vi "Begin.vi"(8 "error in":errorcluster) -> (0 "error out":errorcluster)   [LabVIEW 2019]
doc: "Called before other user functions, this VI is expected to open initial I/O refnums, load in file data, and do all program initialization. Notice that the <B>error out</B> terminal is simply used for data flow. Wiring it to other structures or subVIs ensures that this VI runs first."
uses:
  <vilib>/Rock Robotics/SystemInterfaces/i2clib/i2c_bus.ctl
  <vilib>/Rock Robotics/WPI/DriverStation/WPI_DriverStationRobotMode2.ctl
  <vilib>/Rock Robotics/WPI/Joystick/WPI_JoystickDeviceEnum.ctl
  <vilib>/Rock Robotics/WPI/Solenoid/WPI_SolenoidChannel.ctl
  <vilib>/Rock Robotics/WPI/SafetyOutput/WPI_SafetyOutputConfigMenu.ctl
  <vilib>/Rock Robotics/WPI/ThirdParty/REV Robotics/SPARK MAX/Typedef/Spark MAX Motor Type.ctl
  <vilib>/Rock Robotics/WPI/ThirdParty/REV Robotics/SPARK MAX/Typedef/Spark MAX Sensor Type.ctl
  <vilib>/Rock Robotics/SystemInterfaces/DIO/FPGA_DIOChannel.ctl
  <vilib>/Rock Robotics/SystemInterfaces/DIO/FPGA_DIOPWMChannel.ctl
  Robot Global Data.vi
  <vilib>/Rock Robotics/Network Tables/NT Write String Array.vi
  <vilib>/Rock Robotics/WPI/RobotDrive/WPI_RobotDriveOpen2MotorWithExistingMotors.vi
  <vilib>/Rock Robotics/WPI/Solenoid/WPI_SolenoidOpenDouble.vi
  <vilib>/Rock Robotics/WPI/MotorControl/WPI_MotorControlOpen SPARK.vi
  <vilib>/Rock Robotics/WPI/RobotDrive/WPI_RobotDriveOpen2MotorWithVictorSPX.vi
  <vilib>/Rock Robotics/SystemInterfaces/spilib/spi_bus.ctl
  <vilib>/Rock Robotics/WPI/Gyro/WPI_GyroXRS450_SPI_Open.vi
panel:
  out "String":string="Velocity Tune"
  out "String 2":string="Smart Motion Tune"
  out "String 3":string="Tuning Instructions:\n\n0) Before using this function, you should understand from your specific mechanism the max acceleration and the max velocity. You can obtain these either by design constraints, or running in open loop mode and calculating these values.\n\n1) Set the 'Mode' switch to 'Velocity Tune'\n\n2) Tune the mechanism as you would a Velocity PID loop until the mechanism is controlled fairly well. In this mode the Setpoint slider controls the Velocity of the mechanism.\n\n3) Configure the smart motion parameters, and set the 'Mode' switch to 'Smart Motion'. In this mode, the Setpoint slider controls the Position of the mechansim. For initial tests it is recommended to keep the max velocity and max acceleration lower than the max value, and slowly increase these to the desired level.\n\n4) Test the mechanism by setting the position within the allowable range of the mechanism, and slowly increase limits until the system is working as intended."
  in  "I2C Bus":T1
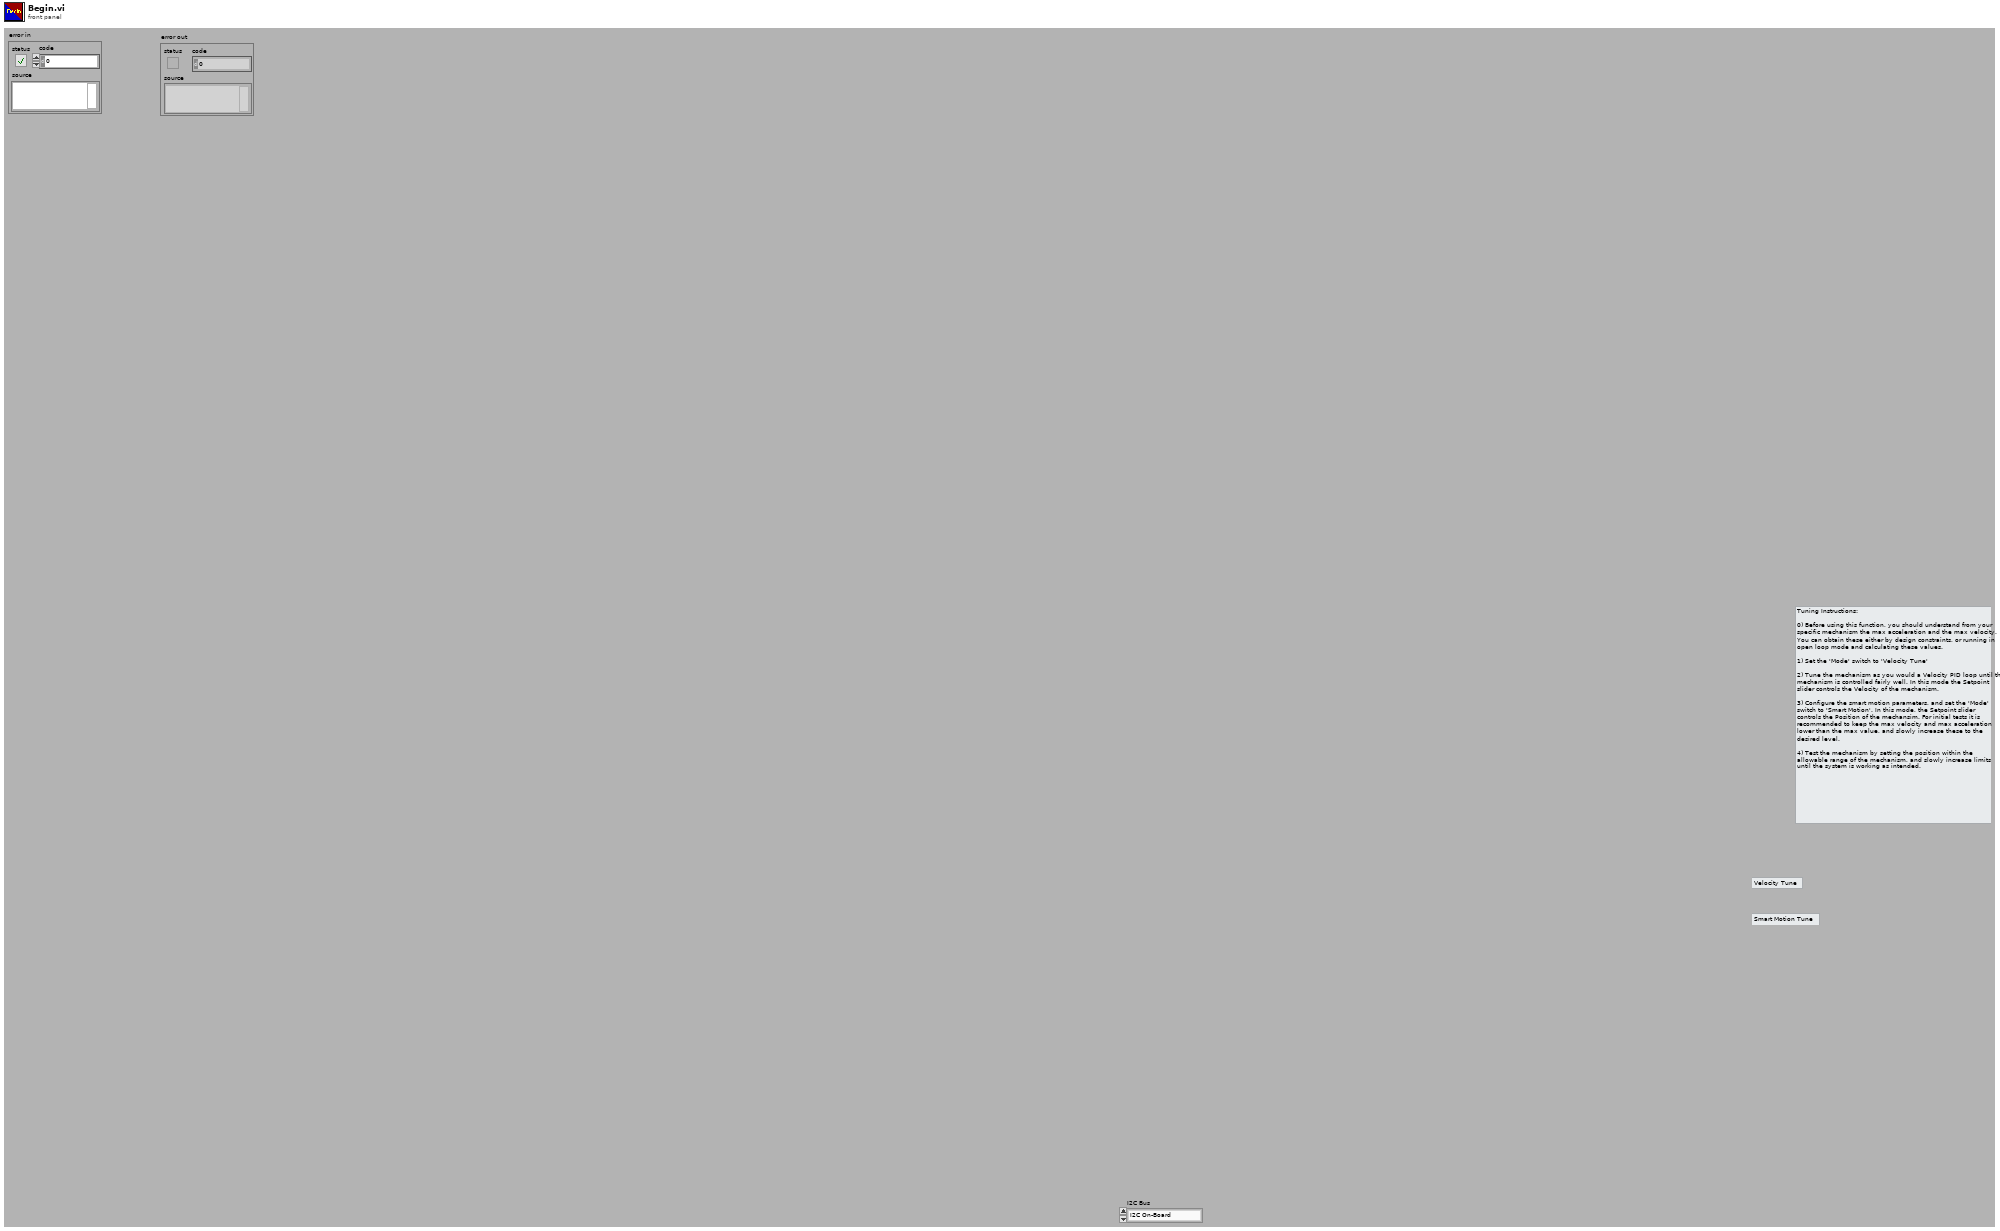
[diagram p1: front panel]
types:
  T1 = typedef "i2c_bus.ctl" = enum16{"I2C On-Board", "I2C MXP", "Invalid"}
  T2 = typedef "FPGA_DIOPWMChannel.ctl" = enum8{"PWM 0", "PWM 1", "PWM 2", "PWM 3", "PWM 4", "PWM 5", "PWM 6", "PWM 7", "PWM 8", "PWM 9", "PWM MXP 0", "PWM MXP 1", "PWM MXP 2", "PWM MXP 3", "PWM MXP 4", "PWM MXP 5", "PWM MXP 6", "PWM MXP 7", "PWM MXP 8", "PWM MXP 9", "Invalid"}
  T3 = typedef "WPI_SafetyOutputConfigMenu.ctl" = enum16{"Enable", "Disable"}
  T4 = typedef "WPI_SolenoidChannel.ctl" = enum8{"Solenoid 0", "Solenoid 1", "Solenoid 2", "Solenoid 3", "Solenoid 4", "Solenoid 5", "Solenoid 6", "Solenoid 7", "Invalid"}
  T5 = typedef "FPGA_DIOChannel.ctl" = enum8{"DIO 0", "DIO 1", "DIO 2", "DIO 3", "DIO 4", "DIO 5", "DIO 6", "DIO 7", "DIO 8", "DIO 9", "DIO MXP 0", "DIO MXP 1", "DIO MXP 2", "DIO MXP 3", "DIO MXP 4", "DIO MXP 5", "DIO MXP 6", "DIO MXP 7", "DIO MXP 8", "DIO MXP 9", "DIO MXP 10", "DIO MXP 11", "DIO MXP 12", "DIO MXP 13", "DIO MXP 14", "DIO MXP 15", "SPI Port CS1", "SPI Port CS2", "SPI Port CS3", "SPI Port MISO", "SPI Port MOSI", "Invalid"}
  T6 = typedef "Spark MAX Sensor Type.ctl" = enum16{"No Sensor", "Hall Sensor", "Encoder", "-Not Available-", "Analog", "Alternate Encoder"}
  T7 = typedef "Spark MAX Motor Type.ctl" = enum16{"Brushed", "Brushless"}
  T8 = typedef "WPI_JoystickDeviceEnum.ctl" = enum16{"USB 0", "USB 1", "USB 2", "USB 3", "USB 4", "USB 5"}
  T9 = typedef "WPI_DriverStationRobotMode2.ctl" = enum16{"Autonomous Disabled", "Autonomous Enabled", "Teleop Disabled", "Teleop Enabled", "Disconnected", "Finish", "Test Disabled", "Test Enabled", "Emergency Stopped"}
  T10 = typedef "WPI_MotorControlDeviceRef.ctl" = cluster{"DeviceStatus":errorcluster, "Type":T11, "PWM":cluster{"PWM Channel":T2, "DeadBand":T12}, "CAN":cluster{"Device Number":u8, "SetOutput VI Ref":variant, "GetOutput VI Ref":variant, "Enable VI Ref":variant, "Disable VI Ref":variant, "Data":variant}, "Invert":bool, "DIO PWM":cluster{"PWM \"Enable\" Channel":T2, "DIOChannel":T5, "PWM Rate":dbl}}
  T11 = typedef "WPI_MotorControlType.ctl" = enum16{"PWM", "CAN", "DIO PWM"}
  T12 = typedef "WPI_PWMDeadband.ctl" = cluster{"Name":string, "maxPositivePwm":i32, "minPositivePwm":i32, "centerPwm":i32, "maxNegativePwm":i32, "minNegativePwm":i32, "angularRange":u16}
  T13 = typedef "WPI_JoystickDevRef.ctl" = cluster{"Device":T8}
  T14 = typedef "WPI_RobotDriveDevRef.ctl" = cluster{"DevStatus":errorcluster, "Motors[]":T10[], "Square Inputs":bool, "Max Output":dbl}
  T15 = typedef "WPI_DigitalInputDevRef.ctl" = cluster{"DevStatus":errorcluster, "DIO Channel":T5}
  T16 = typedef "spi_bus.ctl" = enum16{"SPI On-Board, CS0", "SPI On-Board, CS1", "SPI On-Board, CS2", "SPI On-Board, CS3", "SPI MXP", "Invalid"}
  T17 = typedef "WPI_GyroDevRef.ctl" = cluster{"DevStatus":errorcluster, "Analog Channel":T18, "Gain (VoltsPerDegree/Second)":dbl, "Gyro Type":enum16{"Analog", "XRS450"}, "Handle":i32, "SPI Bus":T16, "Device Found":bool, "Sample Rate":dbl, "Calibrate On Open":bool, "Offset":dbl}
  T18 = typedef "FPGA_AIChannel.ctl" = enum8{"AI 0", "AI 1", "AI 2", "AI 3", "AI MXP 0", "AI MXP 1", "AI MXP 2", "AI MXP 3", "Invalid"}
  T19 = typedef "Color Sensor V3 DevRef.ctl" = cluster{"I2CDevRef":T20}
  T20 = typedef "WPI_I2CDevRef.ctl" = cluster{"DevStatus":errorcluster, "Device Address":u8, "Handle":i32, "I2C Bus":T1}
  T21 = typedef "WPI_SolenoidDevRef.ctl" = cluster{"DevStatus":errorcluster, "Pneumatics Control Module":u8, "Forward Solenoid Channel":T4, "Reverse Solenoid Channel":T4}
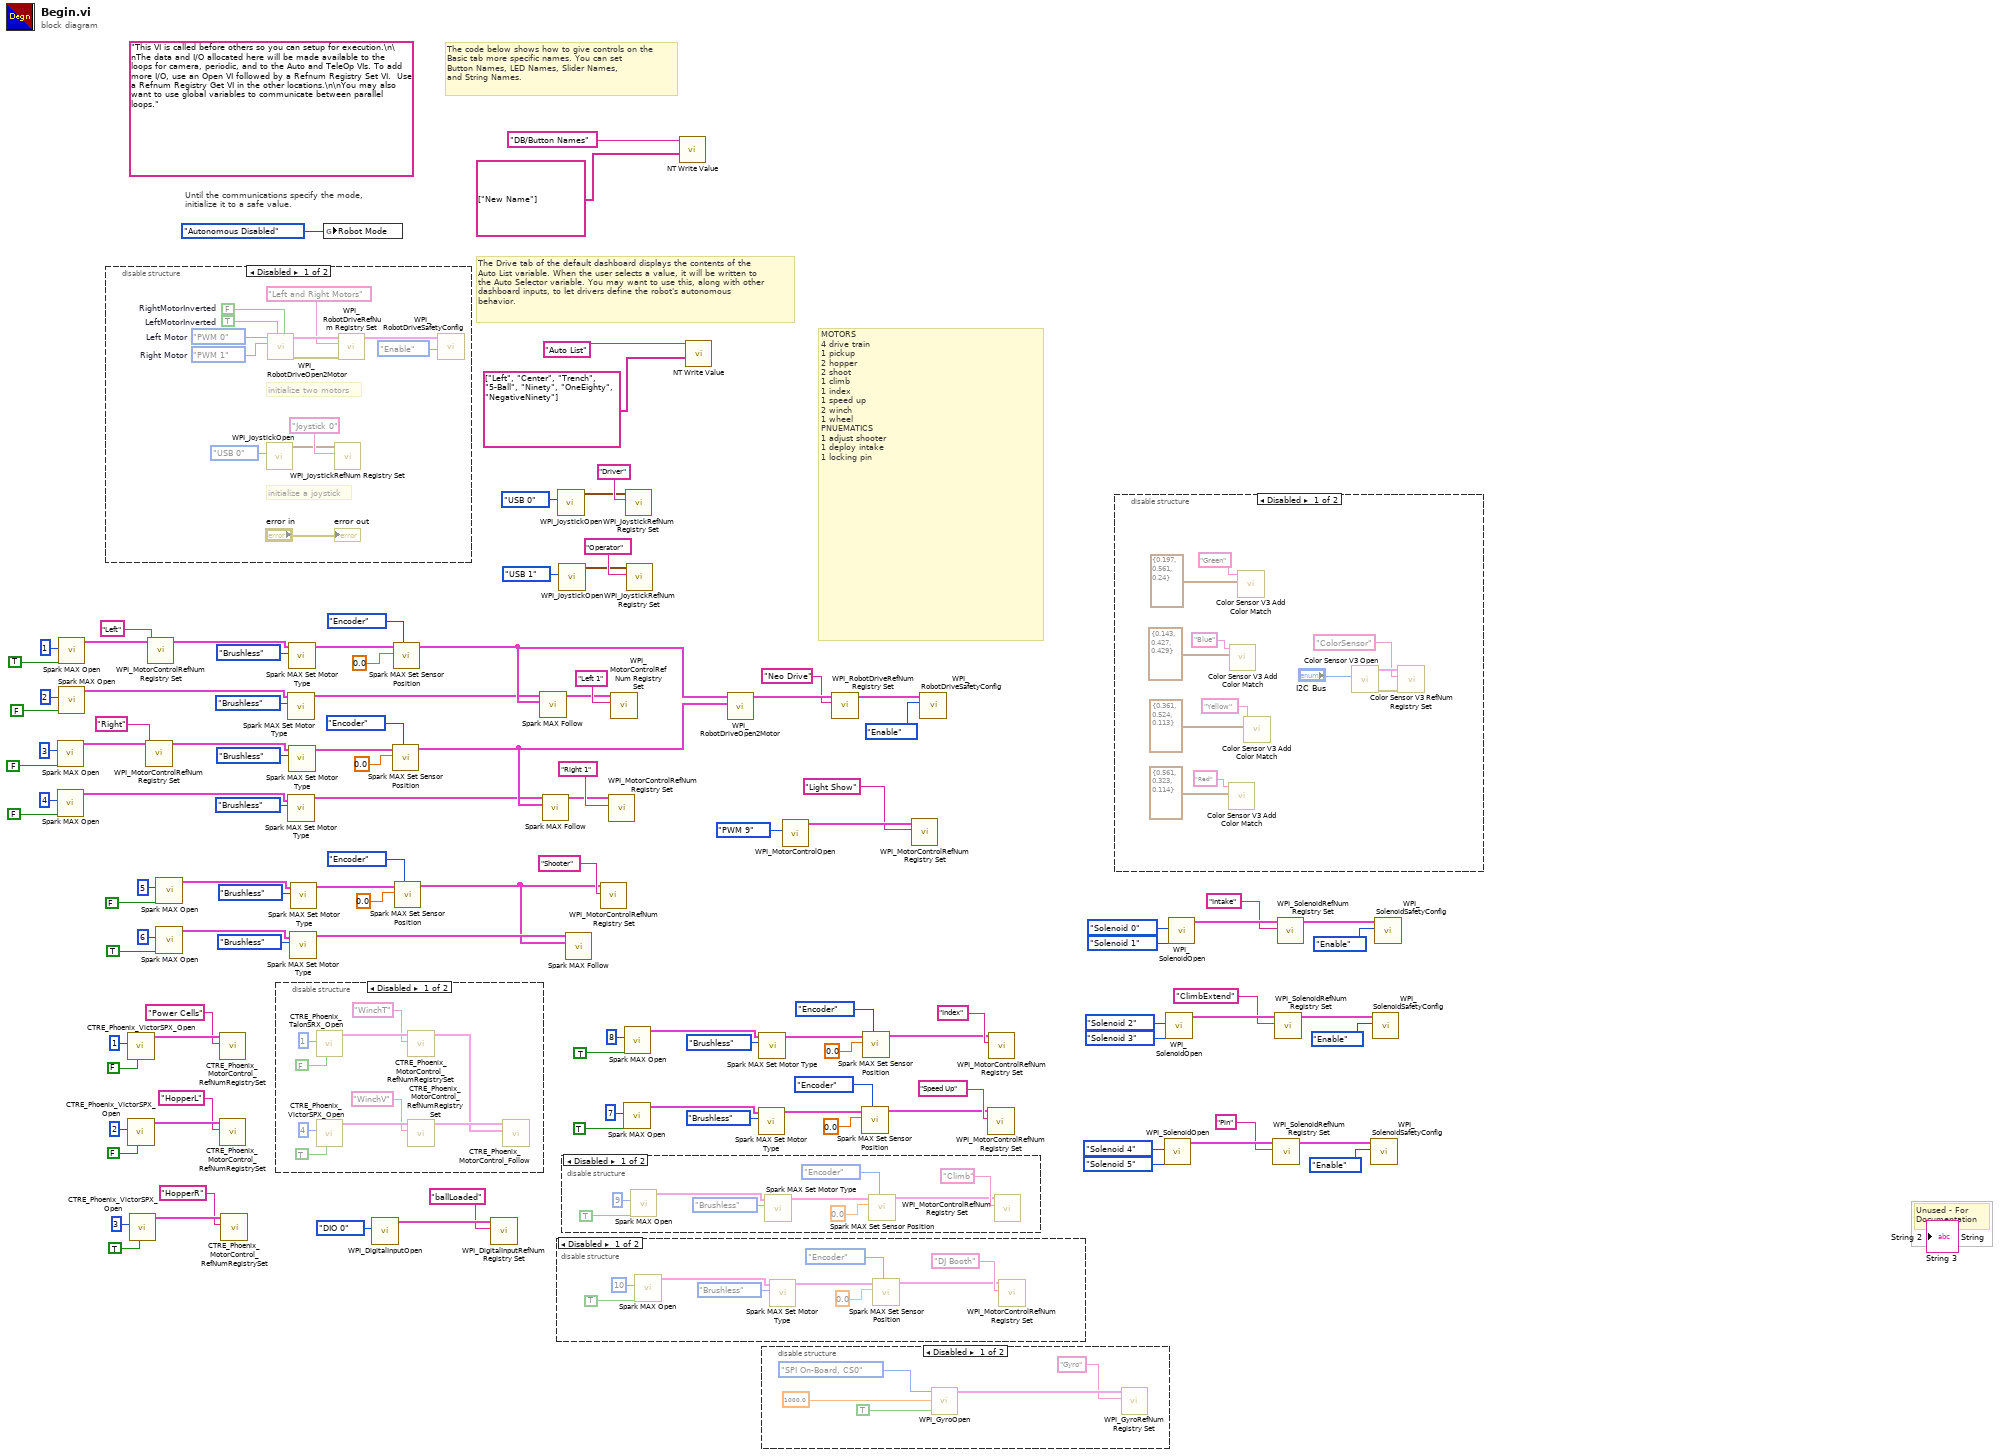
[diagram p0: block diagram]
diagram:
  (unwired) "This VI is called before others so you can setup for execution.\n\nThe data and I/O allocated here will be made available to the loops for camera, periodic, and to the Auto and TeleOp VIs. To add more I/O, use an Open VI followed by a Refnum Registry Set VI.  Use a Refnum Registry Get VI in the other locations.\n\nYou may also want to use global variables to communicate between parallel loops."
  # "Unused - For Documentation"
  # "MOTORS\n4 drive train\n1 pickup\n2 hopper\n2 shoot\n1 climb\n1 index\n1 speed up\n2 winch\n1 wheel\nPNUEMATICS\n1 adjust shooter\n1 deploy intake\n1 locking pin"
  # "The Drive tab of the default dashboard displays the contents of the\nAuto List variable. When the user selects a value, it will be written to\nthe Auto Selector variable. You may want to use this, along with other\ndashboard inputs, to let drivers define the robot's autonomous\nbehavior."
  # "The code below shows how to give controls on the\nBasic tab more specific names. You can set\nButton Names, LED Names, Slider Names,\nand String Names."
  # "Until the communications specify the mode,\ninitialize it to a safe value."
  n1 = call <vilib>:"Spark MAX Open.vi"("Invert"=FALSE, "Device Number"=u8 3) -> ("MotorControlDeviceRef"=w59:T10)  [unwired: 8 in, 1 out]
  n2 = call <vilib>:"Spark MAX Open.vi"("Invert"=FALSE, "Device Number"=u8 4) -> ("MotorControlDeviceRef"=w93:T10)  [unwired: 8 in, 1 out]
  n3 = call <vilib>:"Spark MAX Open.vi"("Invert"=TRUE, "Device Number"=u8 1) -> ("MotorControlDeviceRef"=w62:T10)  [unwired: 8 in, 1 out]
  n4 = call <vilib>:"Spark MAX Open.vi"("Invert"=FALSE, "Device Number"=u8 2) -> ("MotorControlDeviceRef"=w94:T10)  [unwired: 8 in, 1 out]
  n5 = disable-structure shown="Disabled" {
    frame Disabled {
      w124 = FPGA_DIOPWMChannel."PWM 1"  # Right Motor
      w125 = FPGA_DIOPWMChannel."PWM 0"  # Left Motor
      w129 = TRUE  # LeftMotorInverted
      w130 = FALSE  # RightMotorInverted
      # "initialize a joystick"
      # "initialize two motors"
      n6 = call <vilib>:"WPI_JoystickOpen.vi"("JoystickDevice"=WPI_JoystickDeviceEnum."USB 0") -> ("JoystickDevRef"=w120:T13)  [unwired: 10 in]
      n7 = call-poly <vilib>:"WPI_RobotDriveOpen2Motor.vi"("Right Motor Inverted"=w130, "Left Motor Inverted"=w129, "Right Motor"=w124, "Left Motor"=w125) -> ("error out"=w126:errorcluster, "RobotDriveDevRef"=w128:T14)  [unwired: 1 in, 5 out]
      n8 = call <vilib>:"WPI_JoystickRefNum Registry Set.vi"("refnum name"="Joystick 0", "JoystickDevRef"=w120) -> ()  [unwired: 8 in, 2 out]
      n9 = call <vilib>:"WPI_RobotDriveRefNum Registry Set.vi"("error in (no error)"=w126, "refnum name"="Left and Right Motors", "RobotDriveDevRef"=w128) -> ("RobotDriveDevRef"=w123:T14)  [unwired: 1 in, 7 out]
      n10 = call <vilib>:"WPI_RobotDriveSafetyConfig.vi"("mode"=WPI_SafetyOutputConfigMenu."Enable", "RobotDriveDevRef"=w123) -> ()  [unwired: 8 in, 2 out]
      "error out" <- "error in"
    }
    frame Enabled {
    }
  }
  n11 = call <vilib>:"CTRE_Phoenix_VictorSPX_Open.vi"("Invert"=FALSE, "Device Number"=u8 1) -> ("CAN Talon SRX Ref"=w49:T10)  [unwired: 8 in, 1 out]
  n12 = call <vilib>:"CTRE_Phoenix_VictorSPX_Open.vi"("Invert"=FALSE, "Device Number"=u8 2) -> ("CAN Talon SRX Ref"=w42:T10)  [unwired: 8 in, 1 out]
  n13 = call <vilib>:"CTRE_Phoenix_VictorSPX_Open.vi"("Invert"=TRUE, "Device Number"=u8 3) -> ("CAN Talon SRX Ref"=w45:T10)  [unwired: 8 in, 1 out]
  n14 = call <vilib>:"WPI_MotorControlRefNum Registry Set.vi"("refnum name"="Right", "MotorControlDevRef"=w59) -> ("MotorControlDevRef"=w57:T10)  [unwired: 8 in, 1 out]
  n15 = call <vilib>:"WPI_MotorControlRefNum Registry Set.vi"("refnum name"="Left", "MotorControlDevRef"=w62) -> ("MotorControlDevRef"=w60:T10)  [unwired: 8 in, 1 out]
  n16 = call <vilib>:"Spark MAX Open.vi"("Invert"=FALSE, "Device Number"=u8 5) -> ("MotorControlDeviceRef"=w74:T10)  [unwired: 8 in, 1 out]
  n17 = call <vilib>:"Spark MAX Open.vi"("Invert"=TRUE, "Device Number"=u8 6) -> ("MotorControlDeviceRef"=w73:T10)  [unwired: 8 in, 1 out]
  n18 = call <vilib>:"CTRE_Phoenix_MotorControl_RefNumRegistrySet.vi"("refnum name"="Power Cells", "PhoenixMotorControlDevRef"=w49) -> ()  [unwired: 8 in, 2 out]
  n19 = call <vilib>:"CTRE_Phoenix_MotorControl_RefNumRegistrySet.vi"("refnum name"="HopperL", "PhoenixMotorControlDevRef"=w42) -> ()  [unwired: 8 in, 2 out]
  n20 = call <vilib>:"CTRE_Phoenix_MotorControl_RefNumRegistrySet.vi"("refnum name"="HopperR", "PhoenixMotorControlDevRef"=w45) -> ()  [unwired: 8 in, 2 out]
  n21 = disable-structure shown="Disabled" {
    frame Disabled {
      n22 = call <vilib>:"CTRE_Phoenix_TalonSRX_Open.vi"("Invert"=FALSE, "Device Number"=u8 1) -> ("CAN Talon SRX Ref"=w135:T10)  [unwired: 8 in, 1 out]
      n23 = call <vilib>:"CTRE_Phoenix_VictorSPX_Open.vi"("Invert"=TRUE, "Device Number"=u8 4) -> ("CAN Talon SRX Ref"=w139:T10)  [unwired: 8 in, 1 out]
      n24 = call <vilib>:"CTRE_Phoenix_MotorControl_RefNumRegistrySet.vi"("refnum name"="WinchT", "PhoenixMotorControlDevRef"=w135) -> ("PhoenixMotorControlDevRef"=w131:T10)  [unwired: 8 in, 1 out]
      n25 = call <vilib>:"CTRE_Phoenix_MotorControl_RefNumRegistrySet.vi"("refnum name"="WinchV", "PhoenixMotorControlDevRef"=w139) -> ("PhoenixMotorControlDevRef"=w132:T10)  [unwired: 8 in, 1 out]
      n26 = call <vilib>:"CTRE_Phoenix_MotorControl_Follow.vi"("Master Controller to Follow"=w131, "PhoenixMotorControlDevRef"=w132) -> ()  [unwired: 8 in, 2 out]
    }
    frame Enabled {
    }
  }
  n27 = call <vilib>:"Spark MAX Set Motor Type.vi"("Motor Type"=Spark_MAX_Motor_Type."Brushless", "MotorControlDevRef"=w94) -> ("MotorControlDeviceRef"=w63:T10)  [unwired: 8 in, 1 out]
  n28 = call <vilib>:"Spark MAX Set Motor Type.vi"("Motor Type"=Spark_MAX_Motor_Type."Brushless", "MotorControlDevRef"=w93) -> ("MotorControlDeviceRef"=w66:T10)  [unwired: 8 in, 1 out]
  n29 = call <vilib>:"Spark MAX Set Motor Type.vi"("Motor Type"=Spark_MAX_Motor_Type."Brushless", "MotorControlDevRef"=w60) -> ("MotorControlDeviceRef"=w88:T10)  [unwired: 8 in, 1 out]
  n30 = call <vilib>:"Spark MAX Set Motor Type.vi"("Motor Type"=Spark_MAX_Motor_Type."Brushless", "MotorControlDevRef"=w57) -> ("MotorControlDeviceRef"=w89:T10)  [unwired: 8 in, 1 out]
  n31 = call <vilib>:"Spark MAX Set Motor Type.vi"("Motor Type"=Spark_MAX_Motor_Type."Brushless", "MotorControlDevRef"=w73) -> ("MotorControlDeviceRef"=w20:T10)  [unwired: 8 in, 1 out]
  n32 = call <vilib>:"Spark MAX Set Motor Type.vi"("Motor Type"=Spark_MAX_Motor_Type."Brushless", "MotorControlDevRef"=w74) -> ("MotorControlDeviceRef"=w71:T10)  [unwired: 8 in, 1 out]
  n33 = global write "Robot Global Data.vi" "Robot Mode"(WPI_DriverStationRobotMode2."Autonomous Disabled" ("Robot Mode")) -> ()
  n34 = call <vilib>:"WPI_DigitalInputOpen.vi"("DIO Channel"=FPGA_DIOChannel."DIO 0") -> ("DigitalInputDevRef"=w17:T15)  [unwired: 9 in, 1 out]
  n35 = call <vilib>:"Spark MAX Set Sensor Position.vi"("Sensor Type (Hall Sensor)"=Spark_MAX_Sensor_Type."Encoder", "Position"=0.0, "MotorControlDeviceRef"=w89) -> ("MotorControlDeviceRef"=w67:T10)  [unwired: 7 in, 1 out]
  n36 = call <vilib>:"Spark MAX Set Sensor Position.vi"("Sensor Type (Hall Sensor)"=Spark_MAX_Sensor_Type."Encoder", "Position"=0.0, "MotorControlDeviceRef"=w88) -> ("MotorControlDeviceRef"=w64:T10)  [unwired: 7 in, 1 out]
  n37 = call <vilib>:"Spark MAX Set Sensor Position.vi"("Sensor Type (Hall Sensor)"=Spark_MAX_Sensor_Type."Encoder", "Position"=0.0, "MotorControlDeviceRef"=w71) -> ("MotorControlDeviceRef"=w19:T10)  [unwired: 7 in, 1 out]
  n38 = call <vilib>:"WPI_DigitalInputRefNum Registry Set.vi"("refnum name"="ballLoaded", "DigitalInputDevRef"=w17) -> ()  [unwired: 8 in, 2 out]
  n39 = call <vilib>:"Spark MAX Follow.vi"("Master Controller"=w64, "MotorControlDeviceRef"=w63) -> ("MotorControlDeviceRef"=w65:T10)  [unwired: 8 in, 1 out]
  n40 = call <vilib>:"Spark MAX Follow.vi"("Master Controller"=w67, "MotorControlDeviceRef"=w66) -> ("MotorControlDeviceRef"=w68:T10)  [unwired: 8 in, 1 out]
  n41 = disable-structure shown="Disabled" {
    frame Disabled {
      n42 = call <vilib>:"Spark MAX Open.vi"("Invert"=TRUE, "Device Number"=u8 10) -> ("MotorControlDeviceRef"=w146:T10)  [unwired: 8 in, 1 out]
      n43 = call <vilib>:"Spark MAX Set Motor Type.vi"("Motor Type"=Spark_MAX_Motor_Type."Brushless", "MotorControlDevRef"=w146) -> ("MotorControlDeviceRef"=w144:T10)  [unwired: 8 in, 1 out]
      n44 = call <vilib>:"Spark MAX Set Sensor Position.vi"("Sensor Type (Hall Sensor)"=Spark_MAX_Sensor_Type."Encoder", "Position"=0.0, "MotorControlDeviceRef"=w144) -> ("MotorControlDeviceRef"=w141:T10)  [unwired: 7 in, 1 out]
      n45 = call <vilib>:"WPI_MotorControlRefNum Registry Set.vi"("refnum name"="DJ Booth", "MotorControlDevRef"=w141) -> ()  [unwired: 8 in, 2 out]
    }
    frame Enabled {
    }
  }
  n46 = call <vilib>:"WPI_JoystickOpen.vi"("JoystickDevice"=WPI_JoystickDeviceEnum."USB 0") -> ("JoystickDevRef"=w111:T13)  [unwired: 10 in]
  n47 = call <vilib>:"WPI_JoystickOpen.vi"("JoystickDevice"=WPI_JoystickDeviceEnum."USB 1") -> ("JoystickDevRef"=w108:T13)  [unwired: 10 in]
  n48 = disable-structure shown="Disabled" {
    frame Disabled {
      n49 = call <vilib>:"Spark MAX Open.vi"("Invert"=TRUE, "Device Number"=u8 9) -> ("MotorControlDeviceRef"=w155:T10)  [unwired: 8 in, 1 out]
      n50 = call <vilib>:"Spark MAX Set Motor Type.vi"("Motor Type"=Spark_MAX_Motor_Type."Brushless", "MotorControlDevRef"=w155) -> ("MotorControlDeviceRef"=w153:T10)  [unwired: 8 in, 1 out]
      n51 = call <vilib>:"Spark MAX Set Sensor Position.vi"("Sensor Type (Hall Sensor)"=Spark_MAX_Sensor_Type."Encoder", "Position"=0.0, "MotorControlDeviceRef"=w153) -> ("MotorControlDeviceRef"=w150:T10)  [unwired: 7 in, 1 out]
      n52 = call <vilib>:"WPI_MotorControlRefNum Registry Set.vi"("refnum name"="Climb", "MotorControlDevRef"=w150) -> ()  [unwired: 8 in, 2 out]
    }
    frame Enabled {
    }
  }
  n53 = call <vilib>:"Spark MAX Follow.vi"("Master Controller"=w19, "MotorControlDeviceRef"=w20) -> ()  [unwired: 8 in, 2 out]
  n54 = call <vilib>:"WPI_MotorControlRefNum Registry Set.vi"("refnum name"="Shooter", "MotorControlDevRef"=w19) -> ()  [unwired: 8 in, 2 out]
  n55 = call <vilib>:"WPI_MotorControlRefNum Registry Set.vi"("refnum name"="Right 1", "MotorControlDevRef"=w68) -> ()  [unwired: 8 in, 2 out]
  n56 = call <vilib>:"WPI_MotorControlRefNum Registry Set.vi"("refnum name"="Left 1", "MotorControlDevRef"=w65) -> ()  [unwired: 8 in, 2 out]
  n57 = call <vilib>:"Spark MAX Open.vi"("Invert"=TRUE, "Device Number"=u8 7) -> ("MotorControlDeviceRef"=w35:T10)  [unwired: 8 in, 1 out]
  n58 = call <vilib>:"Spark MAX Open.vi"("Invert"=TRUE, "Device Number"=u8 8) -> ("MotorControlDeviceRef"=w26:T10)  [unwired: 8 in, 1 out]
  n59 = call <vilib>:"WPI_JoystickRefNum Registry Set.vi"("refnum name"="Driver", "JoystickDevRef"=w111) -> ()  [unwired: 8 in, 2 out]
  n60 = call <vilib>:"WPI_JoystickRefNum Registry Set.vi"("refnum name"="Operator", "JoystickDevRef"=w108) -> ()  [unwired: 8 in, 2 out]
  n61 = call-poly <vilib>:"NT Write Value.vi"("String Array"=string[] ["New Name"], "Name"="DB/Button Names") -> ()  [unwired: 9 in, 1 out]
  n62 = call-poly <vilib>:"NT Write Value.vi"("String Array"=string[] ["Left", "Center", "Trench", "5-Ball", "Ninety", "OneEighty", "NegativeNinety"], "Name"="Auto List") -> ()  [unwired: 9 in, 1 out]
  n63 = call-poly <vilib>:"WPI_RobotDriveOpen2Motor.vi"("Right Motor Dev Ref"=w67, "Left Motor Dev Ref"=w64) -> ("RobotDriveDevRef"=w84:T14)  [unwired: 8 in, 1 out]
  n64 = call <vilib>:"Spark MAX Set Motor Type.vi"("Motor Type"=Spark_MAX_Motor_Type."Brushless", "MotorControlDevRef"=w35) -> ("MotorControlDeviceRef"=w33:T10)  [unwired: 8 in, 1 out]
  n65 = call <vilib>:"Spark MAX Set Motor Type.vi"("Motor Type"=Spark_MAX_Motor_Type."Brushless", "MotorControlDevRef"=w26) -> ("MotorControlDeviceRef"=w24:T10)  [unwired: 8 in, 1 out]
  n66 = disable-structure shown="Disabled" {
    frame Disabled {
      n67 = call-poly <vilib>:"WPI_GyroOpen.vi"("Calibrate On Open"=TRUE, "Sample Rate (Hz)"=1000.0, "SPI Bus"=spi_bus."SPI On-Board, CS0") -> ("GyroDevRef"=w162:T17)  [unwired: 6 in, 2 out]
      n68 = call <vilib>:"WPI_GyroRefNum Registry Set.vi"("refnum name"="Gyro", "GyroDevRef"=w162) -> ()  [unwired: 8 in, 2 out]
    }
    frame Enabled {
    }
  }
  n69 = call-poly <vilib>:"WPI_MotorControlOpen.vi"("PWM Channel"=FPGA_DIOPWMChannel."PWM 9") -> ("MotorControlDeviceRef"=w2:T10)  [unwired: 9 in, 1 out]
  n70 = call <vilib>:"WPI_RobotDriveRefNum Registry Set.vi"("refnum name"="Neo Drive", "RobotDriveDevRef"=w84) -> ("RobotDriveDevRef"=w82:T14)  [unwired: 8 in, 1 out]
  n71 = call <vilib>:"Spark MAX Set Sensor Position.vi"("Sensor Type (Hall Sensor)"=Spark_MAX_Sensor_Type."Encoder", "Position"=0.0, "MotorControlDeviceRef"=w33) -> ("MotorControlDeviceRef"=w30:T10)  [unwired: 7 in, 1 out]
  n72 = call <vilib>:"Spark MAX Set Sensor Position.vi"("Sensor Type (Hall Sensor)"=Spark_MAX_Sensor_Type."Encoder", "Position"=0.0, "MotorControlDeviceRef"=w24) -> ("MotorControlDeviceRef"=w21:T10)  [unwired: 7 in, 1 out]
  n73 = call <vilib>:"WPI_MotorControlRefNum Registry Set.vi"("refnum name"="Light Show", "MotorControlDevRef"=w2) -> ()  [unwired: 8 in, 2 out]
  n74 = call <vilib>:"WPI_RobotDriveSafetyConfig.vi"("mode"=WPI_SafetyOutputConfigMenu."Enable", "RobotDriveDevRef"=w82) -> ()  [unwired: 8 in, 2 out]
  n75 = call <vilib>:"WPI_MotorControlRefNum Registry Set.vi"("refnum name"="Speed Up", "MotorControlDevRef"=w30) -> ()  [unwired: 8 in, 2 out]
  n76 = call <vilib>:"WPI_MotorControlRefNum Registry Set.vi"("refnum name"="Index", "MotorControlDevRef"=w21) -> ()  [unwired: 8 in, 2 out]
  n77 = disable-structure shown="Disabled" {
    frame Disabled {
      n78 = call <vilib>:"Color Sensor V3 Add Color Match.vi"("Color"=cluster{"R":dbl, "G":dbl, "B":dbl} {"R"=0.561, "G"=0.323, "B"=0.114} ("Red Calibration"), "Name"="Red") -> ()  [unwired: 10 in]
      n79 = call <vilib>:"Color Sensor V3 Add Color Match.vi"("Color"=cluster{"R":dbl, "G":dbl, "B":dbl} {"R"=0.143, "G"=0.427, "B"=0.429} ("Blue Calibration"), "Name"="Blue") -> ()  [unwired: 10 in]
      n80 = call <vilib>:"Color Sensor V3 Add Color Match.vi"("Color"=cluster{"R":dbl, "G":dbl, "B":dbl} {"R"=0.197, "G"=0.561, "B"=0.24} ("Green Calibration"), "Name"="Green") -> ()  [unwired: 10 in]
      n81 = call <vilib>:"Color Sensor V3 Add Color Match.vi"("Color"=cluster{"R":dbl, "G":dbl, "B":dbl} {"R"=0.361, "G"=0.524, "B"=0.113} ("Yellow Calibration"), "Name"="Yellow") -> ()  [unwired: 10 in]
      n82 = call <vilib>:"Color Sensor V3 Open.vi"("I2C Bus"="I2C Bus") -> ("error out"=w166:errorcluster, "ColorSensorDevRef"=w165:T19)  [unwired: 9 in]
      n83 = call <vilib>:"Color Sensor V3 RefNum Registry Set.vi"("error in (no error)"=w166, "refnum name"="ColorSensor", "ColorSensorDevRef"=w165) -> ()  [unwired: 7 in, 2 out]
    }
    frame Enabled {
    }
  }
  n84 = call-poly <vilib>:"WPI_SolenoidOpen.vi"("Reverse Solenoid Channel"=WPI_SolenoidChannel."Solenoid 5", "Forward Solenoid Channel"=WPI_SolenoidChannel."Solenoid 4") -> ("SolenoidDevRef"=w7:T21)  [unwired: 8 in, 1 out]
  n85 = call-poly <vilib>:"WPI_SolenoidOpen.vi"("Reverse Solenoid Channel"=WPI_SolenoidChannel."Solenoid 3", "Forward Solenoid Channel"=WPI_SolenoidChannel."Solenoid 2") -> ("SolenoidDevRef"=w13:T21)  [unwired: 8 in, 1 out]
  n86 = call-poly <vilib>:"WPI_SolenoidOpen.vi"("Reverse Solenoid Channel"=WPI_SolenoidChannel."Solenoid 1", "Forward Solenoid Channel"=WPI_SolenoidChannel."Solenoid 0") -> ("SolenoidDevRef"=w54:T21)  [unwired: 8 in, 1 out]
  n87 = call <vilib>:"WPI_SolenoidRefNum Registry Set.vi"("refnum name"="Pin", "SolenoidDevRef"=w7) -> ("SolenoidDevRef"=w5:T21)  [unwired: 8 in, 1 out]
  n88 = call <vilib>:"WPI_SolenoidRefNum Registry Set.vi"("refnum name"="ClimbExtend", "SolenoidDevRef"=w13) -> ("SolenoidDevRef"=w11:T21)  [unwired: 8 in, 1 out]
  n89 = call <vilib>:"WPI_SolenoidRefNum Registry Set.vi"("refnum name"="Intake", "SolenoidDevRef"=w54) -> ("SolenoidDevRef"=w52:T21)  [unwired: 8 in, 1 out]
  n90 = call <vilib>:"WPI_SolenoidSafetyConfig.vi"("mode"=WPI_SafetyOutputConfigMenu."Enable", "SolenoidDevRef"=w5) -> ()  [unwired: 8 in, 2 out]
  n91 = call <vilib>:"WPI_SolenoidSafetyConfig.vi"("mode"=WPI_SafetyOutputConfigMenu."Enable", "SolenoidDevRef"=w11) -> ()  [unwired: 8 in, 2 out]
  n92 = call <vilib>:"WPI_SolenoidSafetyConfig.vi"("mode"=WPI_SafetyOutputConfigMenu."Enable", "SolenoidDevRef"=w52) -> ()  [unwired: 8 in, 2 out]
